vi "PH_Set.vi"(0 "Device List":T4(array[cluster]), 5 "CFD Settings":T3={"Ch0 Level"=150, "Ch0 ZeroX"=10, "Ch1 Level"=50, "Ch1 ZeroX"=10}, 11 "error in (no error)":errorcluster, 12 "SyncDiv":i32=4, 13 "Offset":i32) -> (3 "pt3 header out":T1={"Comment"="", "RangeNo"=0, "Offset"=0, "AcquisitionTime (ms)"=0, "HardwareSerial"=0, "SyncDivider"=0, "Resolution (ns)"=0.0, "CFD Settings"={"Ch0 Level"=150, "Ch0 ZeroX"=10, "Ch1 Level"=50, "Ch1 ZeroX"=10}, "InpRate0"=0, "InpRate1"=0}, 4 "Router Info":T2(array[cluster]), 6 "Resolution (ps)":i32, 8 "Range":i32, 10 "Count Rate":i32, 15 "error out":errorcluster)   [LabVIEW 2010]
uses:
  PHLib.dll
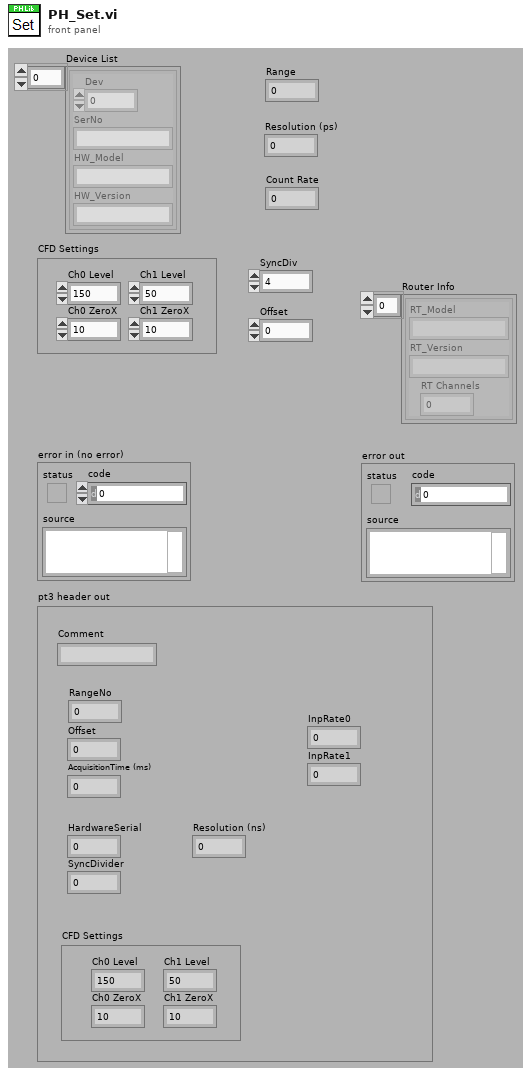
[diagram p1: front panel]
types:
  T1 = cluster{"Comment":string, "RangeNo":i32, "Offset":i32, "AcquisitionTime (ms)":i32, "HardwareSerial":i32, "SyncDivider":i32, "Resolution (ns)":sgl, "CFD Settings":cluster{"Ch0 Level":i32, "Ch0 ZeroX":i32, "Ch1 Level":i32, "Ch1 ZeroX":i32}, "InpRate0":i32, "InpRate1":i32}
  T2 = cluster{"RT_Model":string, "RT_Version":string, "RT Channels":i32}[]
  T3 = cluster{"Ch0 Level":i32, "Ch0 ZeroX":i32, "Ch1 Level":i32, "Ch1 ZeroX":i32}
  T4 = cluster{"Dev":i32, "SerNo":string, "HW_Model":string, "HW_Version":string}[]
  T5 = cluster{"RT_Model":string, "RT_Version":string, "RT Channels":i32}
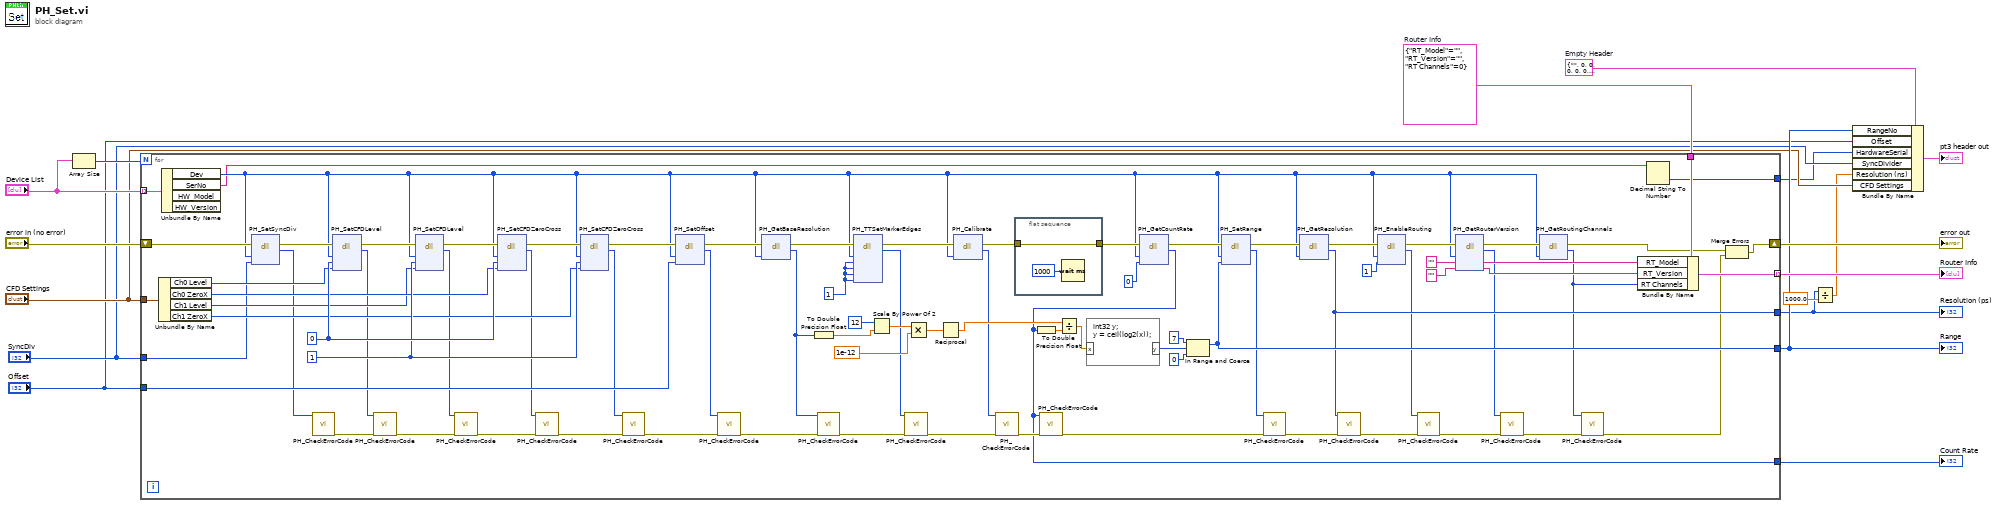
[diagram p0: block diagram]
diagram:
  w10 = T1 {"Comment"="", "RangeNo"=0, "Offset"=0, "AcquisitionTime (ms)"=0, "HardwareSerial"=0, "SyncDivider"=0, "Resolution (ns)"=0.0, "CFD Settings"={"Ch0 Level"=150, "Ch0 ZeroX"=10, "Ch1 Level"=50, "Ch1 ZeroX"=10}, "InpRate0"=0, "InpRate1"=0}  # Empty Header
  w13 = T5 {"RT_Model"="", "RT_Version"="", "RT Channels"=0}  # Router Info
  n1 = Array Size(array="Device List") -> (size(s)=w16:i32)
  n2 = for {
    N: w16 -> [_]
    tunnel: "Device List" -> [w99] mode=indexing
    shift-right: [w22] -> w14
    shift-left: "error in (no error)" -> [w81]
    tunnel: "CFD Settings" -> [w90]
    tunnel: "SyncDiv" -> [w83]
    tunnel: "Offset" -> [w82]
    tunnel: [w65] -> w8
    tunnel: [w31] -> w2
    tunnel: w13 -> [w55]
    tunnel: [w52] -> w12 mode=indexing
    tunnel: [w20] -> w11
    tunnel: [w18] -> w4
    w88 = 1 ("channel")
    w89 = 0 ("channel")
    w91 = 1 ("me3")
    n3 = Unbundle By Name(w90) -> ("Ch0 Level"=w87:i32, "Ch0 ZeroX"=w86:i32, "Ch1 Level"=w85:i32, "Ch1 ZeroX"=w84:i32)
    n4 = Unbundle By Name(w99) -> ("Dev"=w58:i32, "SerNo"=w19:string)  [unwired: 2 out]
    n5 = dll-call lib="C:/LabVIEW Programs/MT Scan PicoHarp/SubVIs/PHLib.dll" fn="PH_SetSyncDiv"(error in=w81, "devidx"=w58, "div"=w83) -> (error out=w98:errorcluster, "return type"=w51:i32)  [unwired: 4 in, 1 out]
    n6 = call "PH_CheckErrorCode.vi"("errcode"=w51) -> ("error out"=w50:errorcluster)  [unwired: 13 in, 1 out]
    n7 = dll-call lib="C:/LabVIEW Programs/MT Scan PicoHarp/SubVIs/PHLib.dll" fn="PH_SetCFDLevel"(error in=w98, "devidx"=w58, "channel"=w89, "value"=w87) -> (error out=w97:errorcluster, "return type"=w49:i32)  [unwired: 5 in, 1 out]
    n8 = call "PH_CheckErrorCode.vi"("errcode"=w49, "error in (no error)"=w50) -> ("error out"=w48:errorcluster)  [unwired: 12 in, 1 out]
    n9 = dll-call lib="C:/LabVIEW Programs/MT Scan PicoHarp/SubVIs/PHLib.dll" fn="PH_SetCFDLevel"(error in=w97, "devidx"=w58, "channel"=w88, "value"=w85) -> (error out=w96:errorcluster, "return type"=w47:i32)  [unwired: 5 in, 1 out]
    n10 = call "PH_CheckErrorCode.vi"("errcode"=w47, "error in (no error)"=w48) -> ("error out"=w45:errorcluster)  [unwired: 12 in, 1 out]
    n11 = dll-call lib="C:/LabVIEW Programs/MT Scan PicoHarp/SubVIs/PHLib.dll" fn="PH_SetCFDZeroCross"(error in=w96, "devidx"=w58, "channel"=w89, "value"=w86) -> (error out=w95:errorcluster, "return type"=w46:i32)  [unwired: 5 in, 1 out]
    n12 = call "PH_CheckErrorCode.vi"("errcode"=w46, "error in (no error)"=w45) -> ("error out"=w43:errorcluster)  [unwired: 12 in, 1 out]
    n13 = dll-call lib="C:/LabVIEW Programs/MT Scan PicoHarp/SubVIs/PHLib.dll" fn="PH_SetCFDZeroCross"(error in=w95, "devidx"=w58, "channel"=w88, "value"=w84) -> (error out=w94:errorcluster, "return type"=w44:i32)  [unwired: 5 in, 1 out]
    n14 = call "PH_CheckErrorCode.vi"("errcode"=w44, "error in (no error)"=w43) -> ("error out"=w41:errorcluster)  [unwired: 12 in, 1 out]
    n15 = dll-call lib="C:/LabVIEW Programs/MT Scan PicoHarp/SubVIs/PHLib.dll" fn="PH_SetOffset"(error in=w94, "devidx"=w58, "offset"=w82) -> (error out=w93:errorcluster, "return type"=w42:i32)  [unwired: 4 in, 1 out]
    n16 = call "PH_CheckErrorCode.vi"("errcode"=w42, "error in (no error)"=w41) -> ("error out"=w40:errorcluster)  [unwired: 12 in, 1 out]
    n17 = dll-call lib="C:/LabVIEW Programs/MT Scan PicoHarp/SubVIs/PHLib.dll" fn="PH_GetBaseResolution"(error in=w93, "devidx"=w58) -> (error out=w92:errorcluster, "return type"=w21:i32)  [unwired: 3 in, 1 out]
    n18 = To Double Precision Float(number=w21) -> (double precision float=w75:dbl)
    n19 = call "PH_CheckErrorCode.vi"("errcode"=w21, "error in (no error)"=w40) -> ("error out"=w39:errorcluster)  [unwired: 12 in, 1 out]
    n20 = dll-call lib="C:/LabVIEW Programs/MT Scan PicoHarp/SubVIs/PHLib.dll" fn="PH_TTSetMarkerEdges"(error in=w92, "devidx"=w58, "me0"=w91, "me1"=w91, "me2"=w91, "me3"=w91) -> (error out=w80:errorcluster, "return type"=w38:i32)  [unwired: 7 in, 1 out]
    n21 = Scale By Power Of 2(n=12, x=w75) -> (x*2^n=w74:dbl)
    n22 = call "PH_CheckErrorCode.vi"("errcode"=w38, "error in (no error)"=w39) -> ("error out"=w37:errorcluster)  [unwired: 12 in, 1 out]
    n23 = Multiply(x=w74, y=1e-12) -> (x*y=w72:dbl)
    n24 = Reciprocal(x=w72) -> (1/x=w67:dbl)
    n25 = dll-call lib="C:/LabVIEW Programs/MT Scan PicoHarp/SubVIs/PHLib.dll" fn="PH_Calibrate"(error in=w80, "devidx"=w58) -> (error out=w79:errorcluster, "return type"=w36:i32)  [unwired: 3 in, 1 out]
    n26 = call "PH_CheckErrorCode.vi"("errcode"=w36, "error in (no error)"=w37) -> ("error out"=w35:errorcluster)  [unwired: 12 in, 1 out]
    n27 = flat-sequence {
      tunnel: w79 -> [w101]
      tunnel: [w101] -> w78
      frame #0 {
        n28 = Wait (ms)(milliseconds to wait=u32 1000) -> ()  [unwired: 1 out]
      }
    }
    n29 = dll-call lib="C:/LabVIEW Programs/MT Scan PicoHarp/SubVIs/PHLib.dll" fn="PH_GetCountRate"(error in=w78, "devidx"=w58, "channel"=0) -> (error out=w70:errorcluster, "return type"=w20:i32)  [unwired: 4 in, 1 out]
    n30 = To Double Precision Float(number=w20) -> (double precision float=w68:dbl)
    n31 = call "PH_CheckErrorCode.vi"("errcode"=w20, "error in (no error)"=w35) -> ("error out"=w33:errorcluster)  [unwired: 12 in, 1 out]
    n32 = Divide(x=w67, y=w68) -> (x/y=w71:dbl)
    n33 = formula code="int32 y;\ny = ceil(log2(x));"("x"=w71) -> ("y"=w66:i32)
    n34 = In Range and Coerce(upper limit=7, x=w66, lower limit=0) -> (coerced(x)=w65:i32)  [unwired: 1 out]
    n35 = dll-call lib="C:/LabVIEW Programs/MT Scan PicoHarp/SubVIs/PHLib.dll" fn="PH_SetRange"(error in=w70, "devidx"=w58, "range"=w65) -> (error out=w69:errorcluster, "return type"=w34:i32)  [unwired: 4 in, 1 out]
    n36 = call "PH_CheckErrorCode.vi"("errcode"=w34, "error in (no error)"=w33) -> ("error out"=w32:errorcluster)  [unwired: 12 in, 1 out]
    n37 = dll-call lib="C:/LabVIEW Programs/MT Scan PicoHarp/SubVIs/PHLib.dll" fn="PH_GetResolution"(error in=w69, "devidx"=w58) -> (error out=w62:errorcluster, "return type"=w31:i32)  [unwired: 3 in, 1 out]
    n38 = call "PH_CheckErrorCode.vi"("errcode"=w31, "error in (no error)"=w32) -> ("error out"=w30:errorcluster)  [unwired: 12 in, 1 out]
    n39 = dll-call lib="C:/LabVIEW Programs/MT Scan PicoHarp/SubVIs/PHLib.dll" fn="PH_EnableRouting"(error in=w62, "devidx"=w58, "enable"=1) -> (error out=w61:errorcluster, "return type"=w27:i32)  [unwired: 4 in, 1 out]
    n40 = call "PH_CheckErrorCode.vi"("errcode"=w27, "error in (no error)"=w30) -> ("error out"=w29:errorcluster)  [unwired: 12 in, 1 out]
    n41 = dll-call lib="C:/LabVIEW Programs/MT Scan PicoHarp/SubVIs/PHLib.dll" fn="PH_GetRouterVersion"(error in=w61, "devidx"=w58, "model"="", "vers"="" ("model")) -> (error out=w60:errorcluster, "return type"=w26:i32, "model"=w54:string, "vers"=w53:string)  [unwired: 3 in, 1 out]
    n42 = call "PH_CheckErrorCode.vi"("errcode"=w26, "error in (no error)"=w29) -> ("error out"=w28:errorcluster)  [unwired: 12 in, 1 out]
    n43 = dll-call lib="C:/LabVIEW Programs/MT Scan PicoHarp/SubVIs/PHLib.dll" fn="PH_GetRoutingChannels"(error in=w60, "devidx"=w58) -> (error out=w24:errorcluster, "return type"=w25:i32)  [unwired: 3 in, 1 out]
    n44 = call "PH_CheckErrorCode.vi"("errcode"=w25, "error in (no error)"=w28) -> ("error out"=w23:errorcluster)  [unwired: 12 in, 1 out]
    n45 = Bundle By Name(cluster=w55, "RT_Model"=w54, "RT_Version"=w53, "RT Channels"=w25) -> (w52:T5)
    n46 = Decimal String To Number(string=w19) -> (number=w18:i32)  [unwired: 2 in, 1 out]
    n47 = Merge Errors(w24, w23) -> (w22:errorcluster)
  }
  "error out" <- w14
  "Range" <- w8
  "Resolution (ps)" <- w2
  "Router Info" <- w12
  "Count Rate" <- w11
  n48 = Divide(x=w2, y=sgl 1000.0) -> (x/y=w1:sgl)
  n49 = Bundle By Name(cluster=w10, "RangeNo"=w8, "Offset"="Offset", "HardwareSerial"=w4, "SyncDivider"="SyncDiv", "Resolution (ns)"=w1, "CFD Settings"="CFD Settings") -> (→"pt3 header out":T1)
